vi "Reset VS Channels.vi"(8 "error in (no error)":errorcluster, 11 "Single Board Loopback in":refnum<class "Single Board Loopback.lvclass">) -> (0 "error out":errorcluster, 3 "Single Board Loopback out":refnum<class "Single Board Loopback.lvclass">)   [LabVIEW 2020]
uses:
  Single Board Loopback/Single Board Loopback.lvclass
  C:/Users/nitest/Desktop/Git 2020/niveristand-custom-device-testing-tools/VeriStandTestCase/VeriStandTestCase.lvclass
  1e32ca70-98be-4c49-9a55-e48adc1a34b6.vi
  <vilib>/NI VeriStand/Execution/Workspace/NI VeriStand - Set Multiple Channel Values.vi
  niveristand-custom-device-testing-tools/VeriStandTestUtilities/VeriStandTestUtilities.lvlib
  <vilib>/NI VeriStand/Execution/Workspace/NI_VS Workspace ExecutionAPI.lvlib
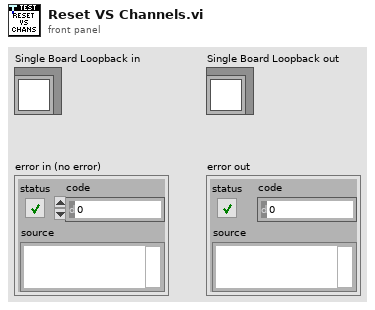
[diagram p1: front panel]
types:
  T1 = typedef "NI_VS Workspace ExecutionAPI.lvlib/WorkspaceAPI.ctl" = refnum<k24>
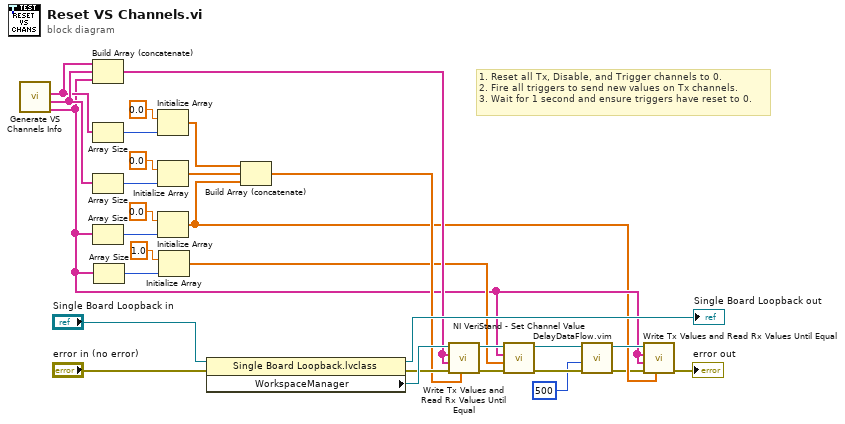
[diagram p0: block diagram]
diagram:
  # "1. Reset all Tx, Disable, and Trigger channels to 0.\n2. Fire all triggers to send new values on Tx channels.\n3. Wait for 1 second and ensure triggers have reset to 0."
  n1 = call "Generate VS Channels Info.vi"() -> ("Tx Trigger Channels Array"=w5:string[], "Tx Disable Channels Array"=w25:string[], "Tx Channels Array"=w24:string[])  [unwired: 7 in, 2 out]
  n2 = Build Array (concatenate)(w24, w25, w5) -> (w14:string[])
  n3 = Array Size(array=w24) -> (size(s)=w17:i32)
  n4 = Array Size(array=w25) -> (size(s)=w21:i32)
  n5 = Array Size(array=w5) -> (size(s)=w20:i32)
  n6 = Array Size(array=w5) -> (size(s)=w8:i32)
  n7 = Initialize Array(0.0 ("element"), w17) -> (w22:dbl[])
  n8 = Initialize Array(0.0 ("element"), w21) -> (w23:dbl[])
  n9 = Initialize Array(0.0 ("element"), w20) -> (w4:dbl[])
  n10 = Initialize Array(1.0 ("element"), w8) -> (w6:dbl[])
  n11 = property class="Single Board Loopback.lvclass"(reference="Single Board Loopback in", error in="error in (no error)") -> (reference out=→"Single Board Loopback out":refnum<class "Single Board Loopback.lvclass">, error out=w15:errorcluster, "WorkspaceManager"=w26:T1)
  n12 = Build Array (concatenate)(w22, w23, w4) -> (w13:dbl[])
  n13 = call "Write Tx Values and Read Rx Values Until Equal.vi"("Tx values"=w13, "error in"=w15, "Rx aliases"=w14, "Tx aliases"=w14, "workspace manager in"=w26) -> ("error out"=w12:errorcluster, "workspace manager out"=w11:T1)  [unwired: 4 in, 1 out]
  n14 = call-poly <vilib>:"NI VeriStand - Set Channel Value.vi"("error in (no error)"=w12, "Values"=w6, "Channels"=w5, "WorkspaceManager in"=w11) -> ("error out"=w10:errorcluster, "WorkspaceManager out"=w9:T1)  [unwired: 6 in]
  n15 = call "DelayDataFlow.vim"("value in"=w10, "milliseconds to wait"=u32 500) -> ("value out"=w3:errorcluster)  [unwired: 2 in, 1 out]
  n16 = call "Write Tx Values and Read Rx Values Until Equal.vi"("Tx values"=w4, "error in"=w3, "Rx aliases"=w5, "Tx aliases"=w5, "workspace manager in"=w9) -> ("error out"=→"error out":errorcluster)  [unwired: 4 in, 2 out]
